vi "Run Measurement.vi"(8 "error in (no error)":errorcluster, 11 "Operator UI in":refnum<class "Server UI.lvclass">) -> (0 "error out":errorcluster, 3 "Operator UI out":refnum<class "Server UI.lvclass">)   [LabVIEW 2026, in "Server UI.lvlib" / "Server UI.lvclass"]
uses:
  Server UI.lvclass
  C:/Users/E2013170/Documents/GitHub/Measurement-Utility-Reference/source/framework/Msmt UI/Measurement UI.lvclass
  C:/Program Files/National Instruments/LabVIEW 2026/vi.lib/ActorFramework/Actor/Actor.lvclass
  Server UI.lvclass/Server UI.ctl
  <vilib>/ActorFramework/Actor/Actor.lvclass/Actor.ctl
  Controller/Messages/Run Measurement Remotely on Client Msg/Run Measurement Remotely on Client Msg.lvclass/Run Measurement Remotely on Client Msg.ctl
  <vilib>/ActorFramework/Message Enqueuer/Message Enqueuer.lvclass/Message Enqueuer.ctl
  Read Connection Showing.vi
  Read Connected Clients.vi
  <vilib>/ActorFramework/Message Enqueuer/Enqueue.vi
  Controller/Messages/Run Measurement Remotely on Client Msg/Run Measurement Remotely on Client Msg.lvclass
  C:/Program Files/National Instruments/LabVIEW 2026/vi.lib/ActorFramework/Message/Message.lvclass
  <vilib>/ActorFramework/Message Priority Queue/Priority Enqueue.vi
  framework/Msmt UI/Measurement UI.lvclass
  <vilib>/ActorFramework/Actor/Actor.lvclass
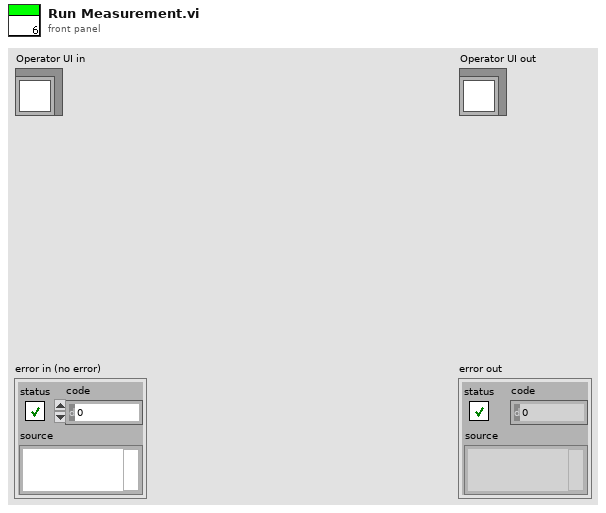
[diagram p1: front panel]
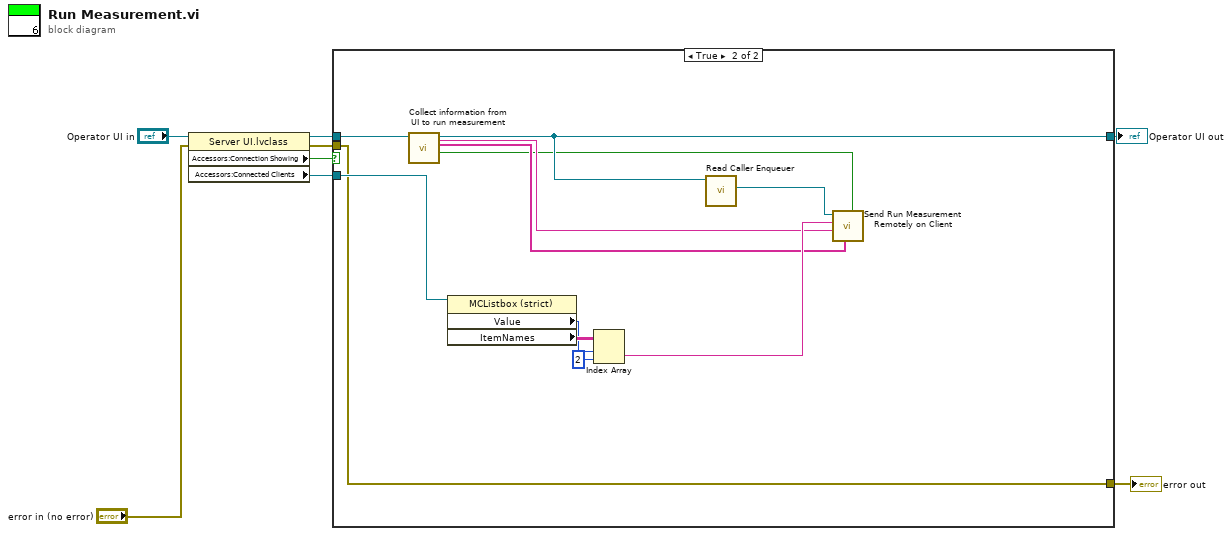
[diagram p0: block diagram]
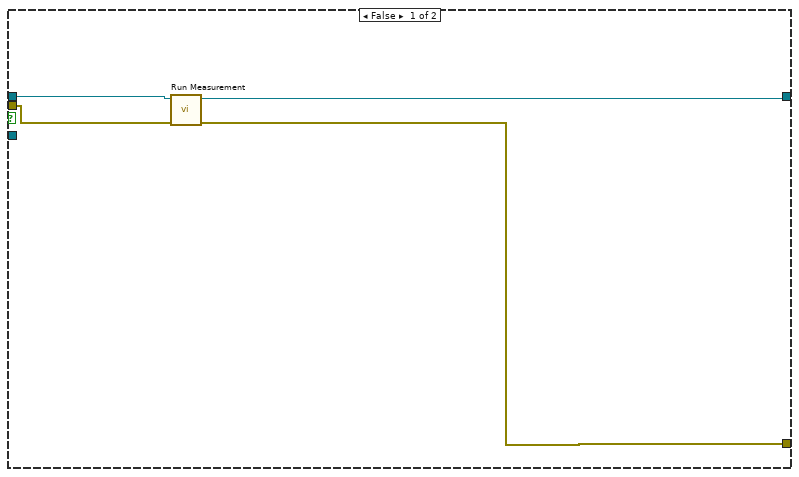
[diagram p2: hidden frame]
diagram:
  n1 = property class="Server UI.lvclass"(reference="Operator UI in", error in="error in (no error)") -> (reference out=w6:refnum<class "Server UI.lvclass">, error out=w4:errorcluster, "Accessors:Connection Showing"=w5:bool, "Accessors:Connected Clients"=w1:refnum<vi>)
  n2 = case shown="True" w5 {
    tunnel: [w11 w20] -> w8
    tunnel: w6 -> [w12 w24]
    tunnel: w4 -> [w10 w15]
    tunnel: [w9 w15] -> w3
    tunnel: w1 -> [_ w23]
    frame False {
      n3 = call-parent "Run Measurement.vi"("error in (no error)"=w10, "Operator UI in"=w12) -> ("error out"=w9:errorcluster, "Operator UI out"=w11:refnum<class "Server UI.lvclass">)  [unwired: 8 in]
    }
    frame True {
      n4 = call "Collect information from UI to run measurement.vi"("Measurement UI in"=w24) -> ("Show UI?"=w14:bool, "Device Names"=w16:string[], "Measurement UI out"=w20:refnum<class "Server UI.lvclass">, "Measurement Name"=w17:string)  [unwired: 3 in, 4 out]
      n5 = property class="MCListbox (strict)"(reference=w23) -> ("Value"=w21:i32, "ItemNames"=w22:string[][])  [unwired: 1 in, 2 out]
      n6 = Index Array(array=w22, index (row)=w21, index (col)=2 ("disabled index (col)")) -> (element=w18:string)
      n7 = call <vilib>:"Read Caller Enqueuer.vi"("Actor"=w20) -> ("Caller Enqueuer"=w19:refnum<class "Message Enqueuer.lvclass">)  [unwired: 10 in]
      n8 = call "Send Run Measurement Remotely on Client.vi"("Show UI?"=w14, "Array of Devices"=w16, "Measurement Name"=w17, "ConnectionID"=w18, "Message Enqueuer"=w19) -> ()  [unwired: 5 in, 2 out]
    }
  }
  "error out" <- w3
  "Operator UI out" <- w8
